vi "Create Path Name.vi"(4 "error in":errorcluster, 7 "filename":string) -> (0 "error out":errorcluster, 3 "path":path)   [LabVIEW 2017, in "File IO.lvclass"]
uses:
  File IO.lvclass
  Global/File Locations.vi
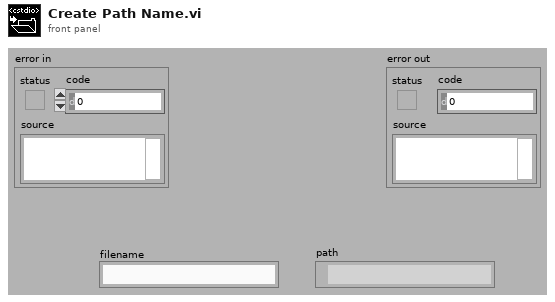
[diagram p1: front panel]
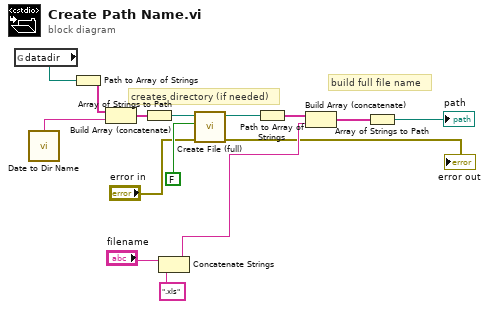
[diagram p0: block diagram]
diagram:
  # "build full file name"
  # "creates directory (if needed)"
  n1 = global read "File Locations.vi" "datadir"() -> (w11:path)
  n2 = call "Date to Dir Name.vi"() -> ("Dir Name"=w13:string)
  n3 = Path to Array of Strings(0:w11) -> (2:w12:string[])  [unwired: 1 out]
  n4 = Build Array (concatenate)(w12, w13) -> (w9:string[])
  n5 = Array of Strings to Path(0:w9) -> (2:w8:path)  [unwired: 1 out]
  n6 = Concatenate Strings("filename", ".xls") -> (w5:string)
  n7 = call "Create File (full).vi"("error in"="error in", "filepath (T)"=FALSE, "pathname"=w8) -> ("error out"=→"error out":errorcluster, "pathOUT"=w7:path)  [unwired: 7 out]
  n8 = Path to Array of Strings(0:w7) -> (2:w6:string[])  [unwired: 1 out]
  n9 = Build Array (concatenate)(w6, w5) -> (w4:string[])
  n10 = Array of Strings to Path(0:w4) -> (2:→"path":path)  [unwired: 1 out]
